vi "json to variant.vi"(8 "error in (no error)":errorcluster, 11 "JSON Value":refnum<class "JSON Value.lvclass">) -> (0 "error out":errorcluster, 3 "Variant":variant)   [LabVIEW 2017, in "JSON Value.lvclass"]
uses:
  JSON Value.lvclass
  subVIs/read variant value.vi
  Array/Get Array Values/Get Array Values (Value[]).vi
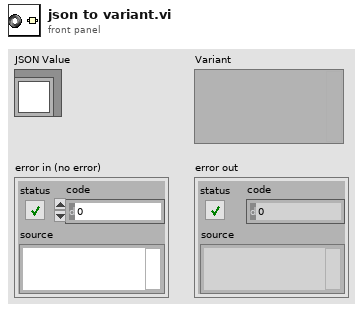
[diagram p1: front panel]
types:
  T1 = typedef "JSON Value.lvclass/JSON Types.ctl" = enum16{"String", "Numeric", "Boolean", "NULL", "Object", "Array"}
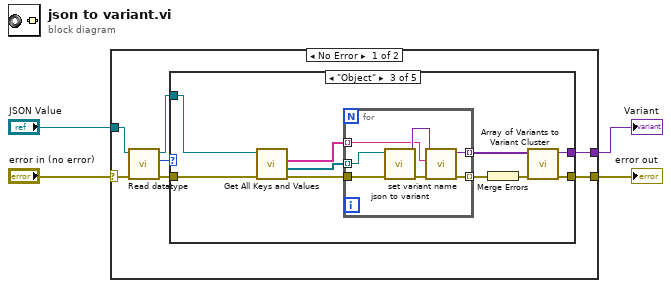
[diagram p0: block diagram]
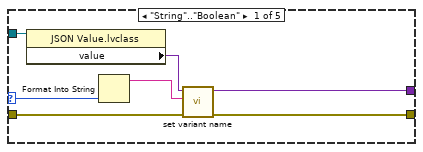
[diagram p2: hidden frame]
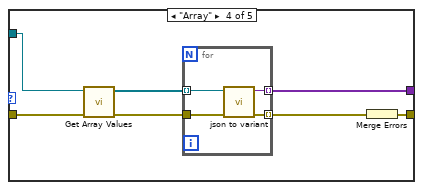
[diagram p4: hidden frame]
diagram:
  n1 = case shown="No Error" "error in (no error)" {
    selector: "error in (no error)" -> [w10 w49]
    tunnel: "JSON Value" -> [w11 _]
    tunnel: [w6 _] -> w2
    tunnel: [w5 w49] -> w1
    frame No Error {
      n2 = call "Read datatype.vi"("error in (no error)"=w10, "JSON Value in"=w11) -> ("error out"=w7:errorcluster, "datatype"=w9:T1, "JSON Value out"=w8:refnum<class "JSON Value.lvclass">)  [unwired: 7 in]
      n3 = case shown="\"Object\"" w9 {
        selector: w9 -> [w13 _ _ _ _]
        tunnel: w8 -> [w18 _ w29 w42 _]
        tunnel: w7 -> [w17 w19 w28 w43 w48]
        tunnel: [w14 _ w22 w39 _] -> w6
        tunnel: [w16 w19 w20 w37 w48] -> w5
        frame "String".."Boolean" {
          n4 = property class="JSON Value.lvclass"(reference=w18) -> ("value"=w15:variant)  [unwired: 1 in, 2 out]
          n5 = Format Into String(w13) -> (resulting string=w12:string)  [unwired: 3 in, 1 out]
          n6 = call "set variant name.vi"("error in (no error)"=w17, "new name"=w12, "variant in"=w15) -> ("error out"=w16:errorcluster, "variant out"=w14:variant)  [unwired: 7 in]
        }
        frame Default {
        }
        frame "Object" {
          n7 = call "Get All Keys and Values.vi"("error in"=w28, "JSON Value in"=w29) -> ("error out"=w25:errorcluster, "values"=w27:refnum<class "JSON Value.lvclass">[], "keys"=w26:string[])  [unwired: 7 in]
          n8 = for {
            tunnel: w27 -> [w36] mode=indexing
            tunnel: w26 -> [w30] mode=indexing
            tunnel: w25 -> [w35]
            tunnel: [w33] -> w24 mode=indexing
            tunnel: [w31] -> w23 mode=indexing
            n9 = call "json to variant.vi"("error in (no error)"=w35, "JSON Value"=w36) -> ("error out"=w34:errorcluster, "Variant"=w32:variant)  [unwired: 8 in]
            n10 = call "set variant name.vi"("error in (no error)"=w34, "new name"=w30, "variant in"=w32) -> ("error out"=w33:errorcluster, "variant out"=w31:variant)  [unwired: 7 in]
          }
          n11 = Merge Errors(w24) -> (w21:errorcluster)
          n12 = call "Array of Variants to Variant Cluster.vi"("error in (no error)"=w21, "Array"=w23) -> ("error out"=w20:errorcluster, "VCluster"=w22:variant)  [unwired: 8 in]
        }
        frame "Array" {
          n13 = call-poly "Get Array Values.vi"("error in (no error)"=w43, "JSON Value in"=w42) -> ("error out"=w40:errorcluster, "values"=w41:refnum<class "JSON Value.lvclass">[])  [unwired: 6 in, 2 out]
          n14 = for {
            tunnel: w41 -> [w47] mode=indexing
            tunnel: w40 -> [w46]
            tunnel: [w45] -> w39 mode=indexing
            tunnel: [w44] -> w38 mode=indexing
            n15 = call "json to variant.vi"("error in (no error)"=w46, "JSON Value"=w47) -> ("error out"=w44:errorcluster, "Variant"=w45:variant)  [unwired: 8 in]
          }
          n16 = Merge Errors(w38) -> (w37:errorcluster)
        }
        frame "NULL" {
        }
      }
    }
    frame Error {
    }
  }
  "error out" <- w1
  "Variant" <- w2
